vi "test_Get Slot Base Module.vi"(8 "error in (no error)":errorcluster, 11 "TestCase in":refnum<class "Scan Engine Scripting API Custom Device Unit Tests.lvclass">) -> (0 "error out":errorcluster, 3 "TestCase out":refnum<class "Scan Engine Scripting API Custom Device Unit Tests.lvclass">)   [LabVIEW 2017, in "Scan Engine Scripting API Custom Device Unit Tests.lvclass"]
uses:
  Scan Engine Scripting API Custom Device Unit Tests.lvclass
  Type Defs/Main Settings.ctl
  Type Defs/Local Chassis Settings.ctl
  Scan Engine Scripting API Custom Device Unit Tests.lvclass/Scan Engine Scripting API Custom Device Unit Tests.ctl
  186bb218-53c3-41f0-9cfc-94fa19d4683d.vi
  Utility/Set Error.vi
  <vilib>/Utility/error.llb/Clear Errors.vi
  Scripting/Utility/Convert Slot Configuration to 9212.vi
  Scripting/Utility/Convert Slot Configuration to 9213.vi
  Scripting/Modules/NI 9475/NI 9475.lvclass
  C:/dev/niveristand-scan-engine-ethercat-custom-device/Custom Device Source/Scripting/Modules/Module/Module.lvclass
  Modules.lvlibp/SD Module/SD Module.lvclass
  C:/dev/niveristand-scan-engine-ethercat-custom-device/Custom Device Source/Modules.lvlibp/RSI Module/RSI Module.lvclass
  Scripting/Modules/NI 9212/NI 9212.lvclass
  Scripting/Modules/NI 9213/NI 9213.lvclass
  Scripting/Modules/NI 9224/NI 9224.lvclass
  Scripting/Modules/NI 9228/NI 9228.lvclass
  Modules.lvlibp/RSI Module/Read Module Page Property.vi
  Modules.lvlibp/RSI Module/Read Model.vi
  Scripting/Utility/Convert Module Model to Module Class.vi
  Modules.lvlibp/SD Module/Read DIO mode.vi
  Modules.lvlibp/RSI Module/Read Channels.vi
  Scripting/Utility/Convert to DI Module.vi
  Scripting/Utility/Convert to DO Module.vi
  Scripting/Utility/Convert to CI PWM Module.vi
  Scripting/Utility/Convert to CDO Module.vi
  Scripting/Utility/Convert to PWM Module.vi
  Globals/Error Strings.vi
  Scripting/Utility/Get Channel Names and Default Values for Slot.vi
  Scripting/Modules/NI 9212/Create NI 9212.vi
  Scripting/Modules/NI 9213/Create NI 9213.vi
  Scripting/Utility/Convert to AI Module.vi
  Scripting/Utility/Convert to AI Vrms Module.vi
  Scripting/Utility/Convert to AI Arms Module.vi
  Scripting/Utility/Convert to DIO Module.vi
  Scripting/Modules/Module/Module.lvclass
  Modules.lvlibp/9212/9212.lvclass
  Modules.lvlibp/9213/9213.lvclass
  Modules.lvlibp/9224/9224.lvclass
  <vilib>/addons/_JKI Toolkits/VI Tester/TestCase.llb/TestCase.lvclass
  Scripting/Scan Engine Scripting.lvlib
  Scan Engine Custom Device.lvlib
  Modules/Module Test Classes/Module Test.lvclass
  C:/Program Files (x86)/National Instruments/LabVIEW 2017/vi.lib/addons/_JKI Toolkits/VI Tester/TestCase.llb/TestCase.lvclass
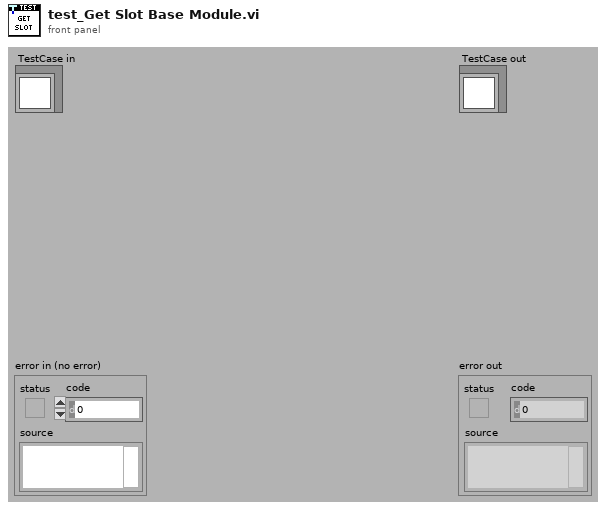
[diagram p1: front panel]
types:
  T1 = typedef "Scan Engine Custom Device.lvlib/Local Chassis Settings.ctl" = cluster{"name":string, "number of slots":i32}
  T2 = typedef "Scan Engine Custom Device.lvlib/Main Settings.ctl" = cluster{"sync to scan":bool, "scan engine decimation":u16, "delay after FPGA load (s)":u16}
  T3 = typedef "Custom Device API.lvlib/Custom Device Item Ref.ctl" = u64
  T4 = typedef "Scan Engine Scripting.lvlib/counter driven output channel settings.ctl" = cluster{"name":string, "default value":bool, "counter driven state":T5}
  T5 = typedef "Scan Engine Scripting.lvlib/Counter Driven Output Channel.lvclass/Counter Driven State.ctl" = enum16{"Disabled", "Enabled"}
  T6 = typedef "Scan Engine Scripting.lvlib/Counter Driven Output Mode.lvclass/Drive from Slot.ctl" = enum16{"Slot 1", "Slot 2", "Slot 3", "Slot 4", "Slot 5", "Slot 6", "Slot 7", "Slot 8"}
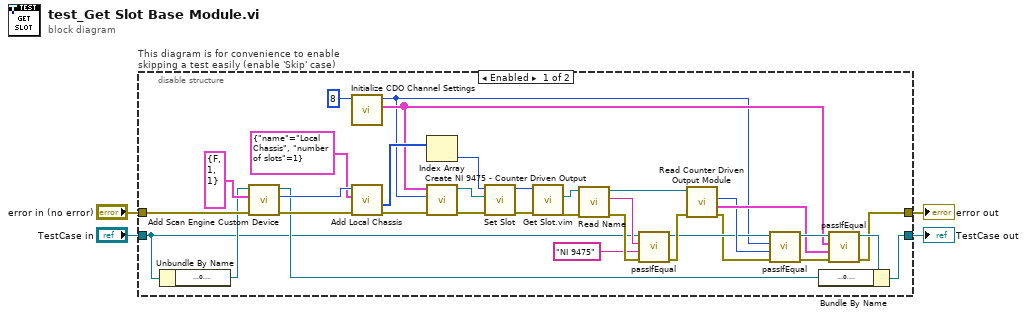
[diagram p0: block diagram]
diagram:
  n1 = disable-structure "This diagram is for convenience to enable skipping a test easily (enable 'Skip' case)" shown="Enabled" {
    disable-tunnel: "TestCase in" -> [w8 w42]
    disable-tunnel: [w28 w40] -> w1
    disable-tunnel: [w14 w41] -> w3
    disable-tunnel: "error in (no error)" -> [w37 w39]
    frame Enabled {
      n2 = Unbundle By Name(w8) -> ("target ref"=w36:refnum<k24>)
      n3 = call "Add Scan Engine Custom Device.vi"("error in"=w37, "settings"=T2 {"sync to scan"=FALSE, "scan engine decimation"=1, "delay after FPGA load (s)"=1}, "target in"=w36) -> ("error out"=w35:errorcluster, "scan engine custom device ref"=w34:T3, "target out"=w22:refnum<k24>)  [unwired: 6 in]
      n4 = call "Initialize CDO Channel Settings.vi"("array size"=8) -> ("channel settings"=w6:T4[], "drive from slot"=w5:T6)  [unwired: 9 in]
      n5 = call "Add Local Chassis.vi"("error in"=w35, "settings"=T1 {"name"="Local Chassis", "number of slots"=1}, "scan engine custom device ref in"=w34) -> ("error out"=w30:errorcluster, "slot refs"=w32:T3[])  [unwired: 4 in, 3 out]
      n6 = Index Array(array=w32) -> (element=w31:T3)  [unwired: 1 in]
      n7 = call "Create NI 9475 - Counter Driven Output.vi"("error in"=w30, "drive from slot"=w5, "channel settings"=w6) -> ("error out"=w29:errorcluster, "NI 9475 out"=w21:refnum<class "NI 9475.lvclass">)  [unwired: 7 in]
      n8 = call "Set Slot.vi"("error in"=w29, "module"=w21, "slot ref in"=w31) -> ("error out"=w20:errorcluster, "slot ref out"=w26:T3)  [unwired: 7 in]
      n9 = call "Get Slot.vim"("error in"=w20, "slot ref in"=w26) -> ("error out"=w17:errorcluster, "module"=w19:refnum<class "Module.lvclass">)  [unwired: 6 in, 2 out]
      n10 = call-dynamic "Read Name.vi"("error in"=w17, "module in"=w19) -> ("error out"=w13:errorcluster, "name"=w11:string, "module out"=w18:refnum<class "Module.lvclass">)  [unwired: 7 in]
      n11 = call-dynamic "passIfEqual.vi"("error in (no error)"=w13, "y"="NI 9475", "x"=w11, "TestCase in"=w8) -> ("error out"=w12:errorcluster, "TestCase out"=w9:refnum<class "Scan Engine Scripting API Custom Device Unit Tests.lvclass">)  [unwired: 6 in]
      n12 = call-dynamic "Read Counter Driven Output Module.vi"("error in"=w12, "module in"=w18) -> ("error out"=w7:errorcluster, "channel settings"=w16:T4[], "drive from slot"=w15:T6)  [unwired: 6 in, 1 out]
      n13 = call-dynamic "passIfEqual.vi"("error in (no error)"=w7, "y"=w15, "x"=w5, "TestCase in"=w9) -> ("error out"=w25:errorcluster, "TestCase out"=w24:refnum<class "Scan Engine Scripting API Custom Device Unit Tests.lvclass">)  [unwired: 6 in]
      n14 = call-dynamic "passIfEqual.vi"("error in (no error)"=w25, "y"=w16, "x"=w6, "TestCase in"=w24) -> ("error out"=w14:errorcluster, "TestCase out"=w23:refnum<class "Scan Engine Scripting API Custom Device Unit Tests.lvclass">)  [unwired: 6 in]
      n15 = Bundle By Name(cluster=w23, "target ref"=w22) -> (w28:refnum<class "Scan Engine Scripting API Custom Device Unit Tests.lvclass">)
    }
    frame Disabled {
      # "skip test result while test is under development"
      n16 = call <vilib>:"skip.vi"("error in (no error)"=w39, "TestCase in"=w42) -> ("error out"=w41:errorcluster, "TestCase out"=w40:refnum<class "Scan Engine Scripting API Custom Device Unit Tests.lvclass">)  [unwired: 8 in]
    }
  }
  "error out" <- w3
  "TestCase out" <- w1
